vi "Fixed-Point Multistage Multirate Filter Modeling and Simulation.vi"() -> ()   [LabVIEW 2023]
doc: "Demonstrates how to use the DFD FXP NStage MRate Modeling VI and the DFD FXP NStage MRate Simulation VI to model and simulate the behavior of a fixed-point multistage multirate filter, respectively."
uses:
  <vilib>/addons/Digital Filter Design/_Objects.llb/DFD Multirate Filtering Mode.ctl
  <vilib>/addons/Digital Filter Design/_Objects.llb/DFD Filter Ripple Specification (Design).ctl
  <vilib>/addons/Digital Filter Design/_Objects.llb/DFD Multirate Filter Specification (Design).ctl
  <vilib>/addons/Digital Filter Design/_Objects.llb/DFD Quantization Settings.ctl
  <vilib>/addons/Digital Filter Design/_Objects.llb/DFD Quantization Sources.ctl
  <vilib>/addons/Digital Filter Design/FXPMRateSim.llb/DFD FXP NStage MRate Simulation (DBL).vi
  <vilib>/addons/Digital Filter Design/Multirate.llb/DFD NStage MRate Filtering (Array).vi
  <vilib>/Analysis/NI_AALBase.lvlib
  <vilib>/addons/Digital Filter Design/NI_DigFilterLicensed.lvlib
  <vilib>/Analysis/NI_AALPro.lvlib
panel:
  out "MSE":dbl format="%.6g"
  out "Error Message":string
  in  "Interstage Word Lengths":i16[](array[numeric])=[16]
  in  "Output Word Length":i16=16
  in  "Input Word Length":i16=16
  out "Filtered Signals":dbl[][](graph)
  in  "Source":enum16{"Sine", "Random Noise"}(ring)=enum."Random Noise"
  in  "Number of Samples":i32=12800
  # "Select Help>>Show Context Help and move the cursor over the VI icon for more information."
  # "Modeling Settings"
  # "Signal Settings"
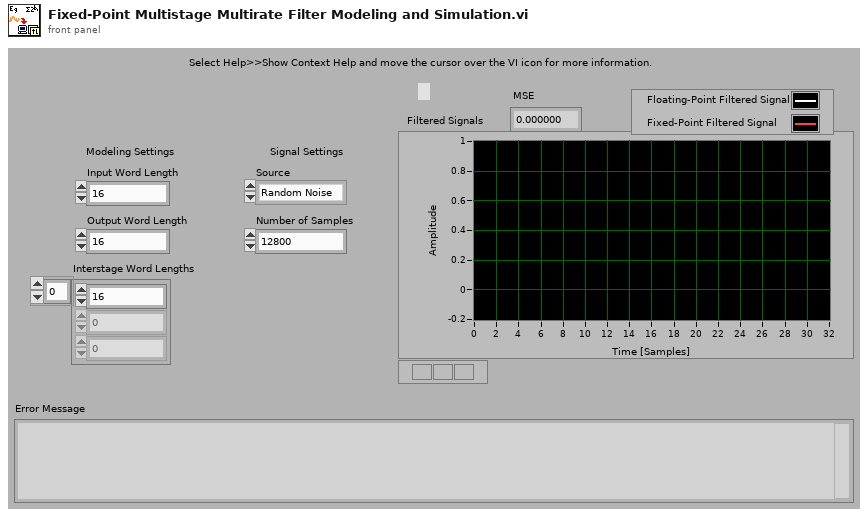
[diagram p1: front panel]
types:
  T1 = typedef "NI_DigFilterLicensed.lvlib/DFD Quantization Settings.ctl" = cluster{"source":T2, "wl":i16, "iwl":i16, "overflow mode":enum16{"Saturation", "Wrap"}, "rounding mode":enum16{"Nearest", "Truncation"}, "signed?":bool}
  T2 = typedef "NI_DigFilterLicensed.lvlib/DFD Quantization Sources.ctl" = u16
  T3 = typedef "NI_DigFilterLicensed.lvlib/DFD Multirate Filter Specification (Design).ctl" = cluster{"fpass":dbl, "fstop":dbl}
  T4 = typedef "NI_DigFilterLicensed.lvlib/DFD Filter Ripple Specification (Design).ctl" = cluster{"passband":dbl, "stopband":dbl, "dB/linear? (T: dB)":bool}
  T5 = typedef "NI_DigFilterLicensed.lvlib/DFD Multirate Filtering Mode.ctl" = u16
  T6 = typedef "NI_DigFilterLicensed.lvlib/DFD Multirate Filter Obj.ctl" = cluster{"mMRate_Structure":enum16{"CIC", "FIR", "IIR", "Lattice"}, "mMRate_Mode":T7, "mMRate_Factor":i32, "mMRate_FIRParams":cluster{"mMRate_FIR_H":dbl[], "mMRate_FIR_IsNyquist?":bool, "mMRate_FIR_IsSymmetric?":bool}, "mMRate_CICParams":cluster{"mMRate_CIC_#Stage":i32, "mMRate_CIC_Lag":i32, "mMRate_CIC_Type":enum16{"Lowpass", "Highpass"}}, "mMRate_Order":i32, "mMRate_Version":string, "mMRate_Comments":string, "mMRate_RationalFactor":cluster{"mMRate_L":i32, "mMRate_M":i32}, "mMRate_Fs":dbl, "mMRate_Quantized?":bool, "mMRate_QFilterGain":dbl, "mMRate_CoefWl":i16, "mMRate_Scaling":cluster{"mMRate_ScaleByPowerOf2?":bool, "mMRate_ScaleType":T8}, "mMRate_InputWl":i16, "mMRate_OutputWl":i16, "mMRate_OutputMode":T9, "mMRate_MultMode":T10, "mMRate_BitPruning":bool, "mMRate_GainWl":i16, "mMRate_OutputFwl":i16, "mMRate_SumIwl":i16, "mMRate_InputIwl ":i16, "mMRate_SumWl":i16, "mMRate_CoefIwl":i16}
  T7 = typedef "NI_DigFilterLicensed.lvlib/DFD Multirate Mode.ctl" = i16
  T8 = typedef "NI_DigFilterLicensed.lvlib/DFD Coef Norm Type.ctl" = enum16{"No Norm", "Time Domain 1-Norm", "Time Domain 2-Norm", "Time Domain Inf-Norm"}
  T9 = typedef "NI_DigFilterLicensed.lvlib/DFD Round-off Mode.ctl" = enum16{"Nearest", "Truncation"}
  T10 = typedef "NI_DigFilterLicensed.lvlib/DFD FXP MRate Multiply Mode.ctl" = enum16{"Truncated", "Full"}
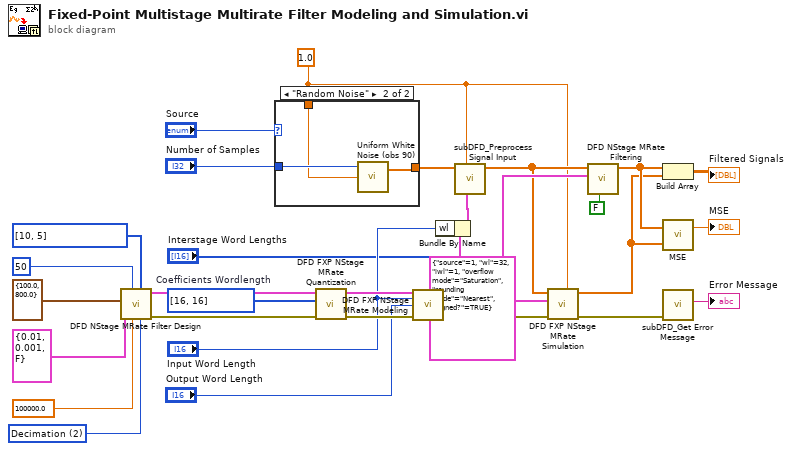
[diagram p0: block diagram]
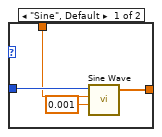
[diagram p2: hidden frame]
diagram:
  w5 = 1.0 ("input range")
  w17 = i16[] [16, 16]  # Coefficients Wordlength
  w19 = T5 2 items=["No Rate Change", "Interpolation", "Decimation"] ("Filtering Mode")
  n1 = call <vilib>:"DFD NStage MRate Filter Design.vi"("filtering mode"=w19, "manual factorization"=i32[] [10, 5] ("Manual Factorization"), "fs in [Hz]"=100000.0 ("Sampling Rate [Hz]"), "factor"=50 ("Factor"), "ripple specs"=T4 {"passband"=0.01, "stopband"=0.001, "dB/linear? (T: dB)"=FALSE} ("Ripple Specs"), "freq specs [Hz]"=T3 {"fpass"=100.0, "fstop"=800.0} ("Freq Spec")) -> ("error out"=w18:errorcluster, "multirate filters out"=w23:T6[])  [unwired: 2 in, 2 out]
  n2 = case shown="\"Random Noise\"" "Source" {
    tunnel: [w33 w35] -> w10
    tunnel: "Number of Samples" -> [w32 w36]
    tunnel: w5 -> [w30 w34]
    frame "Sine", Default {
      n3 = call <vilib>:"Sine Wave.vi"("samples"=w32, "amplitude"=w30, "frequency"=0.001 ("f")) -> ("sine wave"=w33:dbl[])  [unwired: 2 in, 2 out]
    }
    frame "Random Noise" {
      n4 = call <vilib>:"Uniform White Noise (obs 90).vi"("amplitude"=w34, "samples"=w36) -> ("uniform white noise"=w35:dbl[])  [unwired: 1 in, 1 out]
    }
  }
  n5 = call <vilib>:"DFD FXP NStage MRate Quantization.vi"("error in (no error)"=w18, "coefficients word lengths"=w17, "multirate filters in"=w23) -> ("error out"=w15:errorcluster, "multirate filters out"=w16:T6[])  [unwired: 3 in, 4 out]
  n6 = call <vilib>:"DFD FXP NStage MRate Modeling.vi"("interstage word lengths"="Interstage Word Lengths", "output word length"="Output Word Length", "input word length"="Input Word Length", "multirate filters in"=w16) -> ("multirate filters out"=w13:T6[])  [unwired: 4 in, 3 out]
  n7 = Bundle By Name(cluster=T1 {"source"=1, "wl"=32, "iwl"=1, "overflow mode"=enum."Saturation", "rounding mode"=enum."Nearest", "signed?"=TRUE} ("input quantizer"), "wl"="Input Word Length") -> (w7:T1)
  n8 = call <vilib>:"subDFD_Preprocess Signal Input.vi"("input quantizer"=w7, "input range"=w5, "x"=w10) -> ("q[x]"=w9:dbl[])  [unwired: 8 out]
  n9 = call-poly <vilib>:"DFD FXP NStage MRate Simulation.vi"("input range"=w5, "error in (no error)"=w15, "multirate filters"=w13, "signal in"=w9) -> ("error out"=w11:errorcluster, "DBL signal out"=w2:dbl[])  [unwired: 1 in, 5 out]
  n10 = call-poly <vilib>:"DFD NStage MRate Filtering.vi"("zero phase? (T)"=FALSE, "multirate filters"=w13, "signal in"=w9) -> ("signal out"=w3:dbl[])  [unwired: 2 in, 6 out]
  n11 = Build Array(w3, w2) -> (→"Filtered Signals":dbl[][])
  n12 = call <vilib>:"MSE.vi"("X Values"=w2, "Y Values"=w3) -> ("mse"=→"MSE":dbl)  [unwired: 1 out]
  n13 = call <vilib>:"subDFD_Get Error Message.vi"("error in (no error)"=w11) -> ("Error Message"=→"Error Message":string)  [unwired: 10 out]
